vi "Create Pattern Script(Addr).vi"(8 "error in (no error)":errorcluster, 11 "Start_Addr":u16 format="%x") -> (0 "error out":errorcluster, 3 "String":string)   [LabVIEW 2018, in "BML_Frame_Root.lvclass"]
uses:
  BML_Frame_Root.lvclass
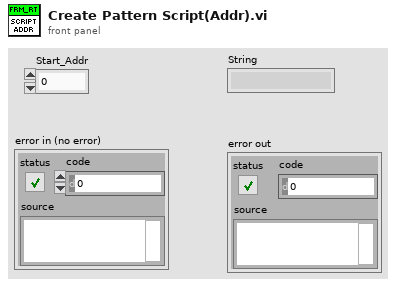
[diagram p1: front panel]
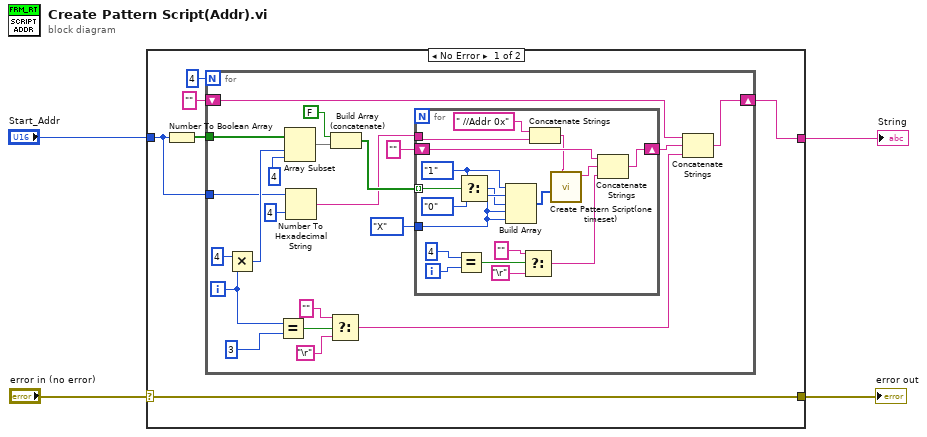
[diagram p0: block diagram]
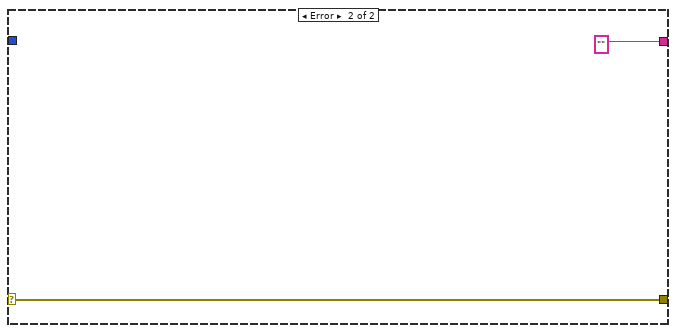
[diagram p2: hidden frame]
diagram:
  n1 = case shown="No Error" "error in (no error)" {
    selector: "error in (no error)" -> [w10 w50]
    tunnel: [w6 ""] -> w3
    tunnel: [w10 w50] -> w2
    tunnel: "Start_Addr" -> [w5 _]
    frame No Error {
      n2 = Number To Boolean Array(number=w5) -> (Boolean array=w9:bool[])
      n3 = for {
        N: 4 -> [_]
        tunnel: w9 -> [w31]
        shift-right: [w16] -> w6
        shift-left: "" -> [w15]
        tunnel: w5 -> [w13]
        i -> [w23]
        n4 = Multiply(x=4 ("y"), y=w23) -> (x*y=w29:i32)
        n5 = Equal?(x=w23, y=3) -> (x = y?=w21:bool)
        n6 = Array Subset(array=w31, index=w29, length=4) -> (w28:bool[])
        n7 = Number To Hexadecimal String(1:i16 4 ("width (-)"), 2:w13) -> (0:w11:string)
        n8 = Select(t="", s=w21, f="\r") -> (s? t:f=w17:string)
        n9 = Build Array (concatenate)(FALSE, w28) -> (w25:bool[])
        n10 = for {
          tunnel: w25 -> [w49] mode=indexing
          shift-right: [w42] -> w18
          shift-left: "" -> [w41]
          tunnel: enum16{"0", "1", "L", "H", "X", "V", "D", "M"}."X" ("element") -> [w37]
          tunnel: w11 -> [w33]
          i -> [w47]
          w36 = enum16{"0", "1", "L", "H", "X", "V", "D", "M"}."1" ("PinState")
          n11 = Equal?(x=4, y=w47) -> (x = y?=w45:bool)
          n12 = Select(t=w36, s=w49, f=enum16{"0", "1", "L", "H", "X", "V", "D", "M"}."0") -> (s? t:f=w35:enum16{"0", "1", "L", "H", "X", "V", "D", "M"})
          n13 = Build Array(w36, w37, w35, w37, w37) -> (w39:enum16{"0", "1", "L", "H", "X", "V", "D", "M"}[])
          n14 = Select(t="", s=w45, f="\r") -> (s? t:f=w40:string)
          n15 = Concatenate Strings(" //Addr 0x" ("Notes"), w33) -> (w32:string)
          n16 = call "Create Pattern Script(one timeset).vi"("Notes"=w32, "PinState"=w39) -> ("string out"=w38:string)  [unwired: 9 in]
          n17 = Concatenate Strings(w41, w38, w40) -> (w42:string)
        }
        n18 = Concatenate Strings(w15, w18, w17) -> (w16:string)
      }
    }
    frame Error {
    }
  }
  "String" <- w3
  "error out" <- w2
